vi "Process Command.vi"(8 "error in (no error)":errorcluster, 10 "user event in":refnum<user-event>, 11 "State in":T1) -> (0 "error out":errorcluster, 3 "State out":T1)   [LabVIEW 2013, in "Connection Handler.lvlib"]
uses:
  Connection Handler.lvlib
  ctl_ClientState.ctl
  <vilib>/Intelligent Energy/Message Queue Helper/ctl_QMH_Message_Typedef.ctl
  ctl_Message.ctl
  <vilib>/Utility/error.llb/DialogType.ctl
  <vilib>/Intelligent Energy/WebSockets API/WebSockets/WebSockets.lvlib
  <vilib>/Intelligent Energy/Message Queue Helper/MessageQueueHelper.lvlib
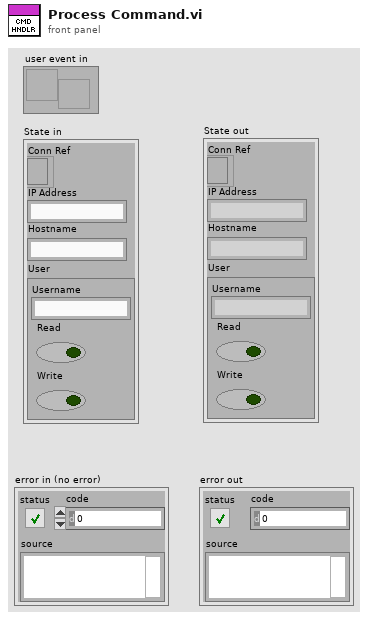
[diagram p1: front panel]
types:
  T1 = typedef "Connection Handler.lvlib/ctl_ClientState.ctl" = cluster{"Conn Ref":refnum<k5>, "IP Address":string, "Hostname":string, "User":cluster{"Username":string, "Read":bool, "Write":bool}}
  T2 = typedef "Connection Handler.lvlib/ctl_Message.ctl" = cluster{"username":string, "message":string}
  T3 = cluster{"command":string, "data":cluster{"session_key":string, "username":string}}
  T4 = typedef "DialogType.ctl" = u16
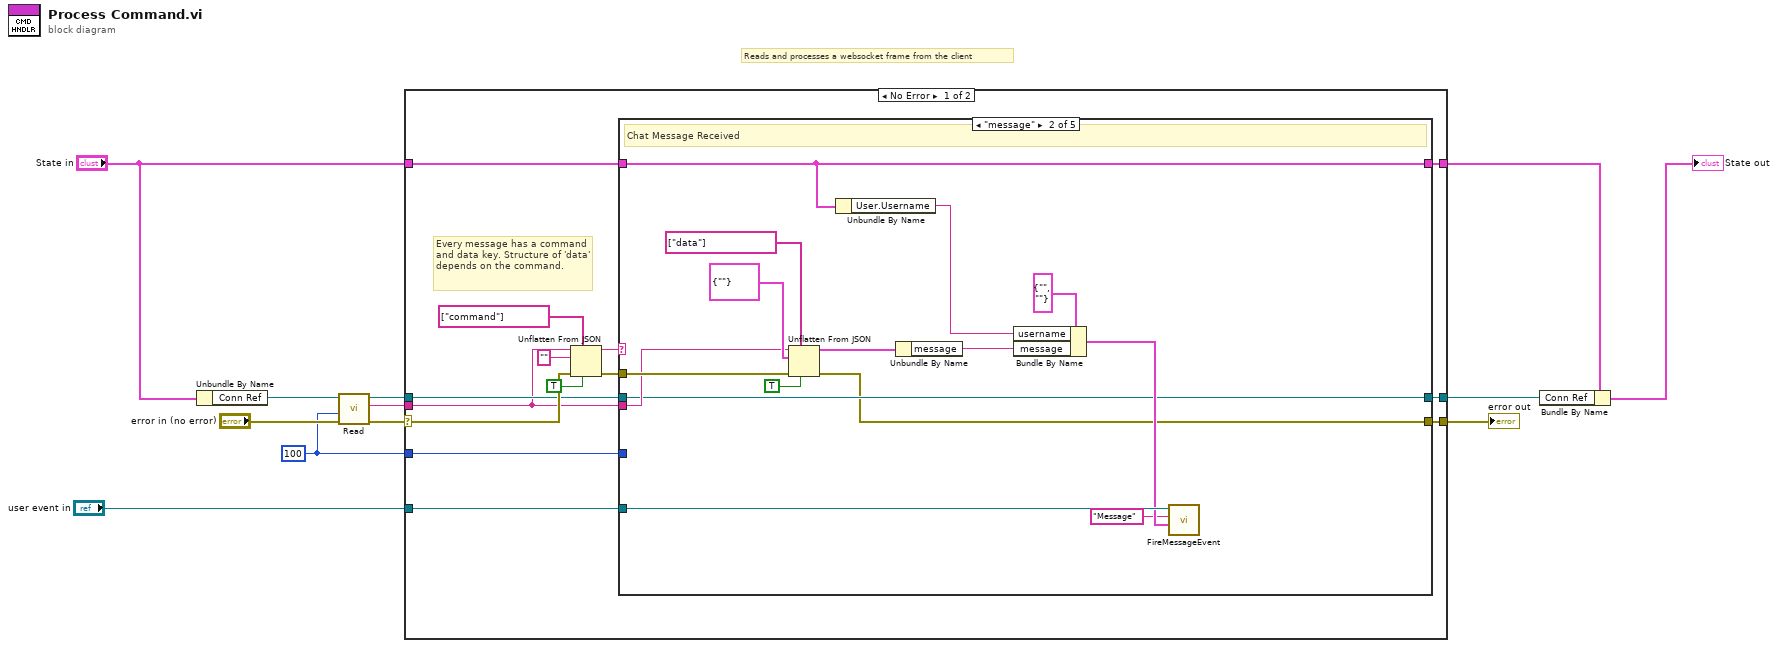
[diagram p0: block diagram]
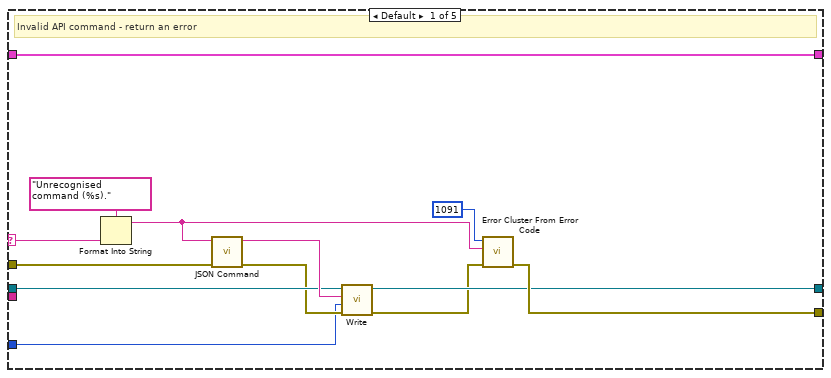
[diagram p2: hidden frame]
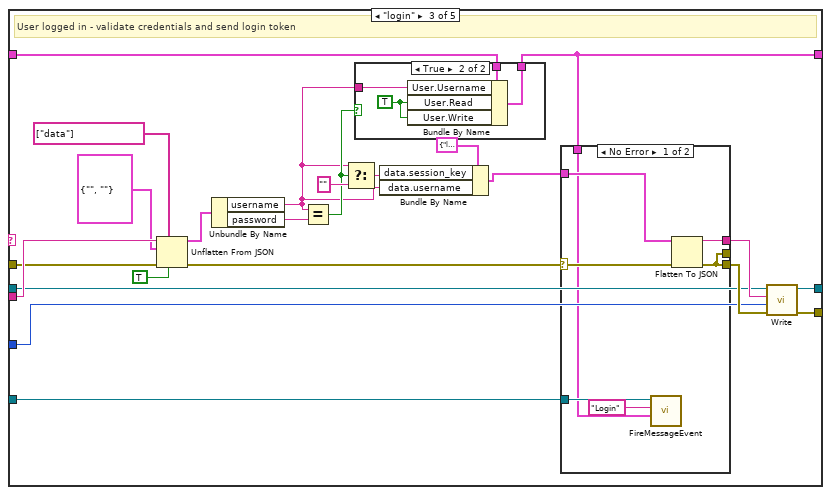
[diagram p3: hidden frame]
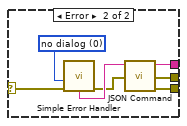
[diagram p5: hidden frame]
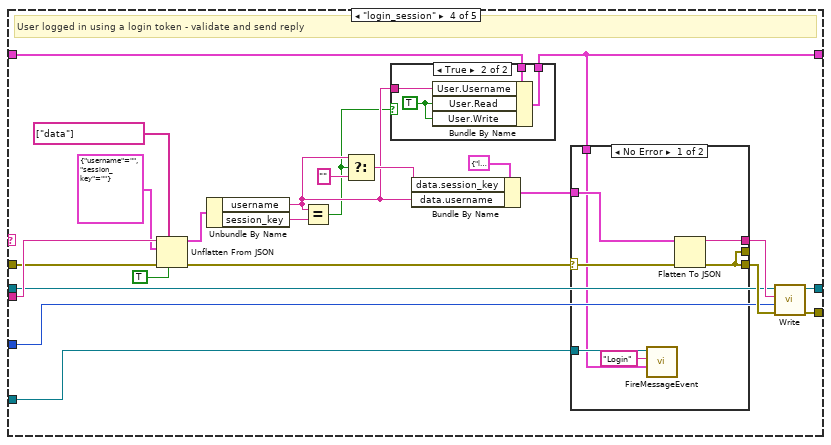
[diagram p6: hidden frame]
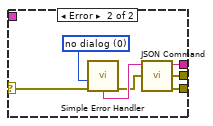
[diagram p8: hidden frame]
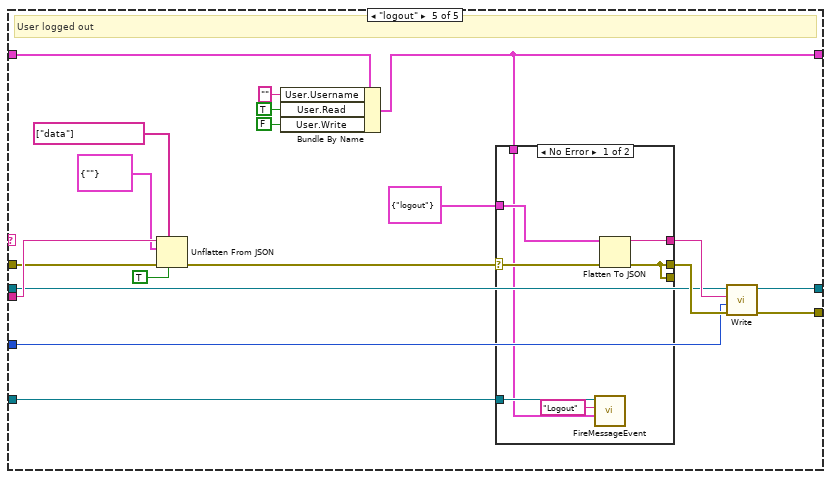
[diagram p9: hidden frame]
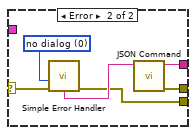
[diagram p10: hidden frame]
diagram:
  w7 = 100 ("timeout ms (5000)")
  # "Reads and processes a websocket frame from the client"
  n1 = Unbundle By Name("State in") -> ("Conn Ref"=w5:refnum<k5>)
  n2 = call <vilib>:"Read.vi"("error in (no error)"="error in (no error)", "timeout ms (5000)"=w7, "WebSocket Connection in"=w5) -> ("error out"=w9:errorcluster, "Data"=w11:string, "WebSocket Connection out"=w8:refnum<k5>)  [unwired: 5 in, 1 out]
  n3 = case shown="No Error" w9 {
    selector: w9 -> [w21 w171]
    tunnel: w11 -> [w18 _]
    tunnel: [w22 w171] -> w10
    tunnel: w8 -> [w20 w170]
    tunnel: [w19 w170] -> w2
    tunnel: w7 -> [w17 _]
    tunnel: "State in" -> [w15 w169]
    tunnel: [w14 w169] -> w4
    tunnel: "user event in" -> [w13 _]
    frame No Error {
      # "Every message has a command and data key. Structure of 'data' depends on the command."
      n4 = Unflatten From JSON(path=string[] ["command"], JSON string=w18, type and defaults="", default null elements? (F)=TRUE, error in (no error)=w21) -> (value=w24:string, error out=w23:errorcluster)  [unwired: 2 in]
      n5 = case shown="\"message\"" w24 {
        selector: w24 -> [w36 _ _ _ _]
        tunnel: w23 -> [w29 w50 w71 w112 w149]
        tunnel: [w39 w40 w74 w115 w152] -> w22
        tunnel: w20 -> [w34 w41 w70 w111 w148]
        tunnel: [w32 w41 w75 w116 w153] -> w19
        tunnel: w18 -> [_ w44 w76 w117 w154]
        tunnel: w17 -> [w28 _ w69 w110 w147]
        tunnel: w15 -> [w27 w48 w58 w100 w142]
        tunnel: [w27 w48 w55 w96 w137] -> w14
        tunnel: w13 -> [_ w54 w56 w97 w138]
        frame Default {
          # "Invalid API command - return an error"
          n6 = Format Into String(format string="Unrecognised command (%s).", w36) -> (resulting string=w33:string)  [unwired: 2 in, 1 out]
          n7 = call "JSON Command.vi"("error in (no error)"=w29, "Error Message"=w33) -> ("error out"=w30:errorcluster, "JSON string"=w35:string)  [unwired: 8 in]
          n8 = call <vilib>:"Write.vi"("error in (no error)"=w30, "timeout ms (5000)"=w28, "Data"=w35, "WebSocket Connection in"=w34) -> ("error out"=w31:errorcluster, "WebSocket Connection out"=w32:refnum<k5>)  [unwired: 6 in]
          n9 = call <vilib>:"Error Cluster From Error Code.vi"("error in (no error)"=w31, "error message (\"\")"=w33, "error code (0)"=1091) -> ("error out"=w39:errorcluster)  [unwired: 6 in]
        }
        frame "message" {
          # "Chat Message Received"
          n10 = Unflatten From JSON(path=string[] ["data"], JSON string=w44, type and defaults=cluster{"message":string} {"message"=""}, default null elements? (F)=TRUE, error in (no error)=w50) -> (value=w43:cluster{"message":string}, error out=w40:errorcluster)  [unwired: 2 in]
          n11 = Unbundle By Name(w48) -> ("User.Username"=w47:string)
          n12 = Unbundle By Name(w43) -> ("message"=w42:string)
          n13 = Bundle By Name(cluster=T2 {"username"="", "message"=""}, "username"=w47, "message"=w42) -> (w46:T2)
          n14 = call <vilib>:"FireMessageEvent.vi"("Data"=w46, "Command"="Message", "User Event in"=w54) -> ()  [unwired: 7 in, 2 out]
        }
        frame "login" {
          # "User logged in - validate credentials and send login token"
          n15 = Unflatten From JSON(path=string[] ["data"], JSON string=w76, type and defaults=cluster{"username":string, "password":string} {"username"="", "password"=""}, default null elements? (F)=TRUE, error in (no error)=w71) -> (value=w66:cluster{"username":string, "password":string}, error out=w63:errorcluster)  [unwired: 2 in]
          n16 = Unbundle By Name(w66) -> ("username"=w57:string, "password"=w62:string)
          n17 = Equal?(x=w57, y=w62) -> (x = y?=w59:bool)
          n18 = Select(t=w57, s=w59, f="") -> (s? t:f=w60:string)
          n19 = case shown="True" w59 {
            tunnel: w58 -> [w78 w82]
            tunnel: [w78 w81] -> w55
            tunnel: w57 -> [_ w80]
            frame False {
            }
            frame True {
              w79 = TRUE ("User.Read")
              n20 = Bundle By Name(cluster=w82, "User.Username"=w80, "User.Read"=w79, "User.Write"=w79) -> (w81:T1)
            }
          }
          n21 = Bundle By Name(cluster=T3 {"command"="login", "data"={"session_key"="", "username"=""}}, "data.session_key"=w60, "data.username"=w57) -> (w64:T3)
          n22 = case shown="No Error" w63 {
            selector: w63 -> [w88 w95]
            tunnel: [w89 w93] -> w73
            tunnel: [w87 w92] -> w72
            tunnel: [w87 w90] -> _
            tunnel: w64 -> [w86 _]
            tunnel: w56 -> [w85 _]
            tunnel: w55 -> [w83 _]
            frame No Error {
              n23 = call <vilib>:"FireMessageEvent.vi"("Data"=w83, "Command"="Login", "User Event in"=w85) -> ()  [unwired: 7 in, 2 out]
              n24 = Flatten To JSON(anything=w86, error in (no error)=w88) -> (JSON string=w89:string, 11:w87:errorcluster)  [unwired: 1 in]
            }
            frame Error {
              w91 = T4 0 items=["no dialog", "OK message", "continue or stop message", "OK message + warnings", "continue/stop + warnings"] ("type of dialog (OK msg:1)")
              n25 = call <vilib>:"Simple Error Handler.vi"("type of dialog (OK msg:1)"=w91, "error in (no error)"=w95) -> ("error out"=w90:errorcluster, "message"=w94:string)  [unwired: 3 in, 3 out]
              n26 = call "JSON Command.vi"("Error Message"=w94) -> ("error out"=w92:errorcluster, "JSON string"=w93:string)  [unwired: 9 in]
            }
          }
          n27 = call <vilib>:"Write.vi"("error in (no error)"=w72, "timeout ms (5000)"=w69, "Data"=w73, "WebSocket Connection in"=w70) -> ("error out"=w74:errorcluster, "WebSocket Connection out"=w75:refnum<k5>)  [unwired: 6 in]
        }
        frame "login_session" {
          # "User logged in using a login token - validate and send reply"
          n28 = Unflatten From JSON(path=string[] ["data"], JSON string=w117, type and defaults=cluster{"username":string, "session_key":string} {"username"="", "session_key"=""}, default null elements? (F)=TRUE, error in (no error)=w112) -> (value=w107:cluster{"username":string, "session_key":string}, error out=w104:errorcluster)  [unwired: 2 in]
          n29 = Unbundle By Name(w107) -> ("username"=w99:string, "session_key"=w103:string)
          n30 = Equal?(x=w99, y=w103) -> (x = y?=w98:bool)
          n31 = Select(t=w99, s=w98, f="") -> (s? t:f=w101:string)
          n32 = case shown="True" w98 {
            tunnel: w100 -> [w119 w123]
            tunnel: [w119 w122] -> w96
            tunnel: w99 -> [_ w121]
            frame False {
            }
            frame True {
              w120 = TRUE ("User.Read")
              n33 = Bundle By Name(cluster=w123, "User.Username"=w121, "User.Read"=w120, "User.Write"=w120) -> (w122:T1)
            }
          }
          n34 = Bundle By Name(cluster=T3 {"command"="login", "data"={"session_key"="", "username"=""}}, "data.session_key"=w101, "data.username"=w99) -> (w105:T3)
          n35 = case shown="No Error" w104 {
            selector: w104 -> [w129 w136]
            tunnel: [w130 w134] -> w114
            tunnel: [w128 w133] -> w113
            tunnel: [w128 w131] -> _
            tunnel: w105 -> [w127 _]
            tunnel: w97 -> [w126 _]
            tunnel: w96 -> [w124 _]
            frame No Error {
              n36 = call <vilib>:"FireMessageEvent.vi"("Data"=w124, "Command"="Login", "User Event in"=w126) -> ()  [unwired: 7 in, 2 out]
              n37 = Flatten To JSON(anything=w127, error in (no error)=w129) -> (JSON string=w130:string, 11:w128:errorcluster)  [unwired: 1 in]
            }
            frame Error {
              w132 = T4 0 items=["no dialog", "OK message", "continue or stop message", "OK message + warnings", "continue/stop + warnings"] ("type of dialog (OK msg:1)")
              n38 = call <vilib>:"Simple Error Handler.vi"("type of dialog (OK msg:1)"=w132, "error in (no error)"=w136) -> ("error out"=w131:errorcluster, "message"=w135:string)  [unwired: 3 in, 3 out]
              n39 = call "JSON Command.vi"("Error Message"=w135) -> ("error out"=w133:errorcluster, "JSON string"=w134:string)  [unwired: 9 in]
            }
          }
          n40 = call <vilib>:"Write.vi"("error in (no error)"=w113, "timeout ms (5000)"=w110, "Data"=w114, "WebSocket Connection in"=w111) -> ("error out"=w115:errorcluster, "WebSocket Connection out"=w116:refnum<k5>)  [unwired: 6 in]
        }
        frame "logout" {
          # "User logged out"
          n41 = Unflatten From JSON(path=string[] ["data"], JSON string=w154, type and defaults=cluster{"username":string} {"username"=""}, default null elements? (F)=TRUE, error in (no error)=w149) -> (error out=w144:errorcluster)  [unwired: 2 in, 1 out]
          n42 = Bundle By Name(cluster=w142, "User.Username"="", "User.Read"=TRUE, "User.Write"=FALSE) -> (w137:T1)
          n43 = case shown="No Error" w144 {
            selector: w144 -> [w161 w168]
            tunnel: [w162 w166] -> w151
            tunnel: [w160 w165] -> w150
            tunnel: [w160 w163] -> _
            tunnel: cluster{"command":string} {"command"="logout"} -> [w159 _]
            tunnel: w138 -> [w158 _]
            tunnel: w137 -> [w156 _]
            frame No Error {
              n44 = call <vilib>:"FireMessageEvent.vi"("Data"=w156, "Command"="Logout", "User Event in"=w158) -> ()  [unwired: 7 in, 2 out]
              n45 = Flatten To JSON(anything=w159, error in (no error)=w161) -> (JSON string=w162:string, 11:w160:errorcluster)  [unwired: 1 in]
            }
            frame Error {
              w164 = T4 0 items=["no dialog", "OK message", "continue or stop message", "OK message + warnings", "continue/stop + warnings"] ("type of dialog (OK msg:1)")
              n46 = call <vilib>:"Simple Error Handler.vi"("type of dialog (OK msg:1)"=w164, "error in (no error)"=w168) -> ("error out"=w163:errorcluster, "message"=w167:string)  [unwired: 3 in, 3 out]
              n47 = call "JSON Command.vi"("Error Message"=w167) -> ("error out"=w165:errorcluster, "JSON string"=w166:string)  [unwired: 9 in]
            }
          }
          n48 = call <vilib>:"Write.vi"("error in (no error)"=w150, "timeout ms (5000)"=w147, "Data"=w151, "WebSocket Connection in"=w148) -> ("error out"=w152:errorcluster, "WebSocket Connection out"=w153:refnum<k5>)  [unwired: 6 in]
        }
      }
    }
    frame Error {
    }
  }
  "error out" <- w10
  n49 = Bundle By Name(cluster=w4, "Conn Ref"=w2) -> (→"State out":T1)
